vi "Array Has Element.vi"(2 "Element":dbl, 3 "Array":dbl[][](array[numeric])) -> (7 "Array has element?":bool)   [LabVIEW 2014]
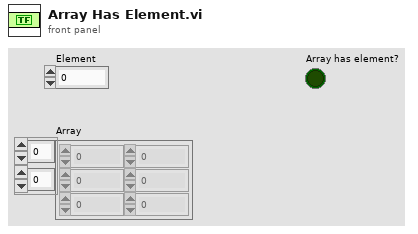
[diagram p1: front panel]
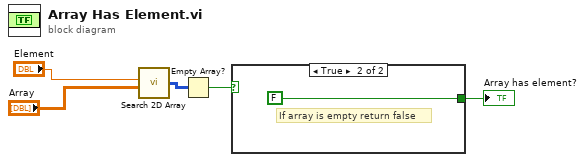
[diagram p0: block diagram]
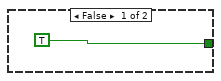
[diagram p2: hidden frame]
diagram:
  n1 = call "Search 2D Array.vi"("Element"="Element", "Array"="Array") -> ("Locations"=w2:i32[][])  [unwired: 5 in]
  n2 = Empty Array?(array=w2) -> (empty?=w1:bool)
  n3 = case shown="True" w1 {
    tunnel: [TRUE FALSE] -> w3
    frame False {
    }
    frame True {
      # "If array is empty return false"
    }
  }
  "Array has element?" <- w3
